vi "Write Last Name.vi"(8 "error in":errorcluster, 10 "Last Name":string, 11 "Person in":refnum<class "Person.lvclass">) -> (0 "error out":errorcluster, 3 "Person out":refnum<class "Person.lvclass">)   [LabVIEW 2020, in "Person.lvclass"]
uses:
  Person.lvclass
  Person.lvclass/Person.ctl
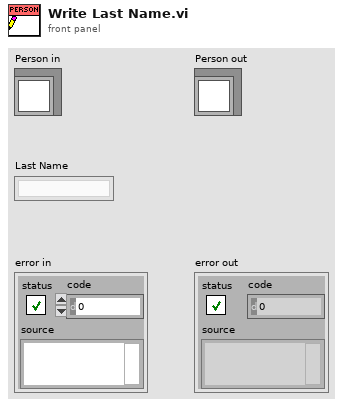
[diagram p1: front panel]
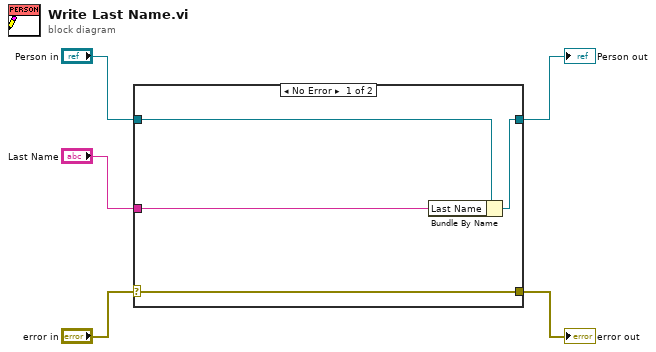
[diagram p0: block diagram]
diagram:
  n1 = case shown="No Error" "error in" {
    selector: "error in" -> [w9 w11]
    tunnel: [w9 w11] -> w4
    tunnel: [w7 w10] -> w2
    tunnel: "Person in" -> [w8 w10]
    tunnel: "Last Name" -> [w6 _]
    frame No Error {
      n2 = Bundle By Name(cluster=w8, "Last Name"=w6) -> (w7:refnum<class "Person.lvclass">)
    }
    frame Error {
    }
  }
  "error out" <- w4
  "Person out" <- w2
